vi "EditorEinfachCRIO-04-02-17.vi"() -> ()   [LabVIEW 2010]
panel:
  in  "Tab Control":T1(tab)
  in  "Dateiordner Housekeeping":path=path "C:/Users/Atmos/Desktop/Johnny"
  in  "Dateiname Housekeeping":string
  in  "DateiordnerECD1":path
  in  "DateinameECD1":string
  in  "DateiordnerECD2":path
  in  "DateinameECD2":string
  in  "Modul1/AI sicherer Bereich":dbl[][](array[numeric])=[[0.0, 0.0, 0.0, 0.0, 0.0, 0.0, 0.0, 0.0, 0.0, 0.0, 0.0, 0.0, 0.0, 0.0, 0.0, 0.0, 0.0, 0.0, 0.0, 0.0, 0.0, 0.0, 0.0, 0.0, 0.0, 0.0, 0.0, 0.0, 0.0, 0.0, 0.0, 0.0]]
  in  "Modul1/AIsNamen":string[](array[string])
  in  "Modul1/AI koeff":dbl[][](array[numeric])=[[0.0, 0.0, 0.0, 0.0, 0.0, 0.0, 0.0, 0.0, 0.0, 0.0, 0.0, 0.0, 0.0, 0.0, 0.0, 0.0, 0.0, 0.0, 0.0, 0.0, 0.0, 0.0, 0.0, 0.0, 0.0, 0.0, 0.0, 0.0, 0.0, 0.0, 0.0, 0.0]]
  in  "AIsNamenZurücksetzen":bool
  in  "Modul2/AIsNamen":string[](array[string])
  in  "Modul2/AI koeff":dbl[][](array[numeric])=[[0.0, 0.0, 0.0, 0.0, 0.0, 0.0, 0.0, 0.0, 0.0, 0.0, 0.0, 0.0, 0.0, 0.0, 0.0, 0.0, 0.0, 0.0, 0.0, 0.0, 0.0, 0.0, 0.0, 0.0, 0.0, 0.0, 0.0, 0.0, 0.0, 0.0, 0.0, 0.0]]
  in  "Modul2/AI sicherer Bereich":dbl[][](array[numeric])=[[0.0, 0.0, 0.0, 0.0, 0.0, 0.0, 0.0, 0.0, 0.0, 0.0, 0.0, 0.0, 0.0, 0.0, 0.0, 0.0, 0.0, 0.0, 0.0, 0.0, 0.0, 0.0, 0.0, 0.0, 0.0, 0.0, 0.0, 0.0, 0.0, 0.0, 0.0, 0.0]]
  in  "Modul3/AIsNamen":string[](array[string])
  in  "Modul3/AI koeff":dbl[][](array[numeric])=[[0.0, 0.0, 0.0, 0.0, 0.0, 0.0, 0.0, 0.0, 0.0, 0.0, 0.0, 0.0, 0.0, 0.0, 0.0, 0.0, 0.0, 0.0, 0.0, 0.0, 0.0, 0.0, 0.0, 0.0, 0.0, 0.0, 0.0, 0.0, 0.0, 0.0, 0.0, 0.0]]
  in  "Modul3/AI sicherer Bereich":dbl[][](array[numeric])=[[0.0, 0.0, 0.0, 0.0, 0.0, 0.0, 0.0, 0.0, 0.0, 0.0, 0.0, 0.0, 0.0, 0.0, 0.0, 0.0, 0.0, 0.0, 0.0, 0.0, 0.0, 0.0, 0.0, 0.0, 0.0, 0.0, 0.0, 0.0, 0.0, 0.0, 0.0, 0.0]]
  out "Schnelle Heizungen":string[](array[string])
  in  "Traps/MachsKoeff":dbl[][](array[numeric])=[[0.0, 0.0, 0.0, 0.0, 0.0, 0.0, 0.0, 0.0, 0.0, 0.0, 0.0, 0.0, 0.0, 0.0, 0.0, 0.0, 0.0, 0.0, 0.0, 0.0, 0.0, 0.0, 0.0, 0.0, 0.0, 0.0, 0.0, 0.0, 0.0, 0.0, 0.0, 0.0]]
  in  "Traps/Machs sicherer Bereich":dbl[][](array[numeric])=[[0.0, 0.0, 0.0, 0.0, 0.0, 0.0, 0.0, 0.0, 0.0, 0.0, 0.0, 0.0, 0.0, 0.0, 0.0, 0.0, 0.0, 0.0, 0.0, 0.0, 0.0, 0.0, 0.0, 0.0, 0.0, 0.0, 0.0, 0.0, 0.0, 0.0, 0.0, 0.0]]
  in  "LangsameHeizungen":string[](array[string])
  in  "ModuleLH":i32[](array[numeric]) min=1 max=3 step=1
  in  "AIsLH":i32[](array[numeric]) min=0 max=31 step=1
  in  "DIOsMod0Name":string[](array[string])
  in  "DIOsMod0Nr":i32[](array[numeric]) min=0 max=63 step=1
  in  "DIOsMod1Name":string[](array[string])
  in  "DIOsMod1Nr":i32[](array[numeric]) min=0 max=63 step=1
  in  "DIOsMod2AName":string[](array[string])
  in  "DIOsMod2ANr":i32[](array[numeric]) min=0 max=63 step=1
  in  "DIOsMod2BName":string[](array[string])
  in  "DIOsMod2BNr":i32[](array[numeric]) min=0 max=63 step=1
  out "AnzahlRegler/Modul":i32[](array[numeric])
  in  "Regler für den Probenfluß":i32
  in  "ReglerNameMod0":string[](array[string])
  in  "ReglerNameMod1":string[](array[string])
  in  "ReglerNameMod2A":string[](array[string])
  in  "ReglerNameMod2B":string[](array[string])
  in  "MWabfragenMod0":string[](array[string])=[":060F0401210120", ":06100401210120", ":06110401210120"]
  in  "MWabfragenMod1":string[](array[string])=[":060F0401210120", ":06100401210120", ":06110401210120"]
  in  "MWabfragenMod2A":string[](array[string])=[":060F0401210120", ":06100401210120", ":06110401210120"]
  in  "MWabfragenMod2B":string[](array[string])=[":060F0401210120", ":06100401210120", ":06110401210120"]
  in  "SPvorgebenMod0":string[](array[string])=[":060F020121", ":0610020121", ":0611020121"]
  in  "SPvorgebenMod1":string[](array[string])=[":060F020121", ":0610020121", ":0611020121"]
  in  "SPvorgebenMod2A":string[](array[string])=[":060F020121", ":0610020121", ":0611020121"]
  in  "SPvorgebenMod2B":string[](array[string])=[":060F020121", ":0610020121", ":0611020121"]
  in  "FaktorMod0":dbl[](array[numeric])=[9.375e-05, 9.375e-05, 9.375e-05]
  in  "FaktorMod1":dbl[](array[numeric])=[9.375e-05, 9.375e-05, 9.375e-05]
  in  "FaktorMod2A":dbl[](array[numeric])=[9.375e-05, 9.375e-05, 9.375e-05]
  in  "FaktorMod2B":dbl[](array[numeric])=[9.375e-05, 9.375e-05, 9.375e-05]
  in  "MWAntwortMod0":string[](array[string])=[":060F020121", ":0610020121", ":0611020121"]
  in  "MWAntwortMod1":string[](array[string])=[":060F020121", ":0610020121", ":0611020121"]
  in  "MWAntwortMod2A":string[](array[string])=[":060F020121", ":0610020121", ":0611020121"]
  in  "MWAntwortMod2B":string[](array[string])=[":060F020121", ":0610020121", ":0611020121"]
  in  "ReglerMod0 sicherer Bereich":dbl[][](array[numeric])=[[9.375e-05, 9.375e-05, 9.375e-05]]
  in  "ReglerMod1 sicherer Bereich":dbl[][](array[numeric])=[[9.375e-05, 9.375e-05, 9.375e-05]]
  in  "ReglerMod2A sicherer Bereich":dbl[][](array[numeric])=[[9.375e-05, 9.375e-05, 9.375e-05]]
  in  "ReglerMod2B sicherer Bereich":dbl[][](array[numeric])=[[9.375e-05, 9.375e-05, 9.375e-05]]
  in  "Metavariablen grüner Bereich":dbl[][](array[numeric])=[[0.0, 0.0, 0.0, 0.0, 0.0, 0.0, 0.0, 0.0, 0.0, 0.0, 0.0, 0.0, 0.0, 0.0, 0.0, 0.0, 0.0, 0.0, 0.0, 0.0, 0.0, 0.0, 0.0, 0.0, 0.0, 0.0, 0.0, 0.0, 0.0, 0.0, 0.0, 0.0]]
  in  "Metavariablen":string[](array[string])
  in  "Startmethode":i32=1
  in  "MethodeLöschen":bool
  in  "MethodeDuplizieren":bool
  out "Methoden":T2(array[cluster]) {"FPGAPID"."proportional gain (Kc)" format="%.11g"; "FPGAPID"."integral gain (Kc*Ts/Ti)" format="%.11g"; "FPGAPID"."derivative gain (Kc*Td/Ts)" format="%.11g"}
  in  "T_MainMach2":dbl[](array[numeric])
  in  "t_MainMach2":dbl[](array[numeric])
  in  "T_MainMach1":dbl[](array[numeric])
  in  "t_MainMach1":dbl[](array[numeric])
  in  "EinstellungenSpeichern":bool
  out "LangsameHeizungen":string[](array[string])
  in  "AllesSpeichern":bool
  in  "Methodenname":string
  in  "Int.Stop2":dbl
  in  "Int.Start2":dbl
  in  "Int.Stop1":dbl
  in  "Int.Start1":dbl
  in  "ZeitpktMS-2":dbl
  in  "ZeitpktMS-1":dbl
  in  "SPMPV":i32[](array[numeric])
  in  "ZeitpunkteMPV":dbl[](array[numeric])
  in  "Wert2":dbl
  in  "Vergleichsoperator2":dbl(ring) items=["<", "<=", "=", ">=", ">", "=/="]
  in  "AbfragbareVariablen2":dbl(ring) items=["T1-Trap1", "T1-Trap2", "T1-StirlingKühlkopf", "T1-PreCol1", "T1-PreCol2", "T1-MainCol1a", "T1-MainCol1b", "T1-MainCol2a", "T1-MainCol2b", "T1-Bronkhorst1a", "T1-Bronkhorst1b", "T1-Bronkhorst2a", "T1-Bronkhorst2b", "T1-2Pos1B", "T1-Spare9", "T1-2Pos1A", "T1-Spare10", "T1-TurboPump", "T1-StirlingPlatine", "T1-Spare5", "T1-Spare6", "T1-Spare7", "T1-Spare8", "F1-MFM1", "F1-MFM0D [mL]", "P1-MethaneHP", "P1-MethaneLP", "P1-Vacuum", "TurboSpeed", "I1-MS-AC", "I1-Trap1", "I1-Trap2", "T2-ECD1a", "T2-ECD1b", "T2-ECD2a", "T2-ECD2b", "T2-Col1a", "T2-Col1b", "T2-Col2a", "T2-Col2b", "T2-Spare1", "T2-Spare2", "T2-Oven_a", "T2-Oven_b", "T2-Spare3", "T2-Spare4", "T2-Spare5", "F2-MFM0", "F2-MFM2A", "F2-MFM2B", "P2-N2O_HP", "P2-N2O_LP", "P2-CO2_HP", "P2-CO2_LP", "AI-Spare1", "FL-MFM1000mL", "AI-Spare3", "AI-Spare4", "StirlingAlarm", "StirlingEmerg.", "AI-Spare7", "AI-Spare8", "AI-Spare9", "FL-MFM30mL", "T0-DC/DC5", "I0-24V_M0", "I0-48V_M1", "I0-24V_M1", "I0-28V_M2", "T0-Spare3", "T0-Spare2", "T0-Spare4", "T0-DC/DC7", "I0-20V_Laptop", "I0-28V_M1", "I0-24V_M2", "I0-12V_Licor", "T0-Spare1", "T0-Drier", "T0-Spare5", "F0-MFM0A [L]", "TL-Licor_a", "P0-Span-HP", "P0-spare1", "P0-Stickstoff-LP", "P0-Helium-LP", "P0-Cal-HP", "P0-P9Tavco[bar]", "F0-MFM0B [L]", "TL-Licor_b", "P0-Span-LP", "P0-spare2", "P0-Stickstoff-HP", "P0-Helium-HP", "P0-Cal-LP", "F0-MFM3", "T-Trap1", "T-Trap2", "T-PreMach1", "T-PreMach2", "T-MainMach1", "T-MainMach2", "PrC0", "PrC0-Licor", "PrC1-Säule2", "PrC1-Säule1", "MFC1-Sample", "MFC1-Methan", "PrC1-BackFlush1", "PrC1-BackFlush2", "MFC2A", "MFC2B", "MFC2C", "PrC2A", "MFC2D", "MFC2E", "PrC2B", "Gesamte Zeit", "Methodenzeit", "Zykluszeit Mod0", "Zykluszeit Mod1", "Zykluszeit Mod2A", "Zykluszeit Mod2B", "PositionMPV", "OverflowB", "OverflowA", "StirlingAlarmAlarm!"]
  in  "Dateien fürs MS schicken?":bool
  in  "Zwangsbedingungen":dbl[][](array[numeric])
  out "ZwangsBedingungen":string[][](array[string])
  in  "löschen":bool
  in  "Bedingung Nr. X":i32
  in  "Bedingung übernehmen":bool
  in  "Ausgangswert":dbl
  in  "BedienbareVariablen":dbl(ring) items=["D0-48V_M1", "D0-28V_M1", "D0-Pump2", "DL-LiCalS1H", "D-Spare2", "D-Spare4", "D0-28V_M2", "D0-Pump1", "D0-S01/EV1", "DL-Licor", "D0-EV3", "D0-EV2", "D1-StopMS", "D1-StartMS", "D1-TrapEvac1", "D1-TrapEvac2", "D1-2Pos1A", "D1-2Pos1B", "D1-TurboPump", "D1-PrePump", "D1-VacPump1", "D1-VacPump2", "D1-Stirling", "D1-P_MS", "D1-S1B(7)", "D1-S1A(6)", "D1-S1G", "D1-Fan3", "D1-LüfterMach1", "D1-LüfterMach2", "D1-MS-Power", "D2-SpülflußA", "D2-2Pos2B", "D2-2Pos2A", "D2-ECD1HeaterOff", "D2-Fan1", "D2-Fan2", "D2-Probe2A", "D2-Probe2B", "D2-SpülflußB", "D2-ECD2HeaterOff", "Servo1 an", "Servo2 an", "Servo1 kalt", "Servo2 kalt", "Heizen?Trap1", "Heizen?Trap2", "Heizen?PreCol1", "Heizen?PreCol2", "Heizen?MainCol1", "Heizen?MainCol2", "SollwertTrap1", "SollwertTrap2", "SollwertPreCol1", "SollwertPreCol2", "SollwertMainCol1", "SollwertMainCol2", "Methodennummer", "STOPP!!!", "H1-Valve1B heizen?", "H1-Bronkhorst1 heizen?", "H1-Bronkhorst2 heizen?", "H1-Valve1A heizen?", "H0-Drier heizen?", "HL-Licor heizen?", "H2-ECD2 heizen?", "H2-Oven heizen?", "H2-Spare1 heizen?", "H2-Col2 heizen?", "H2-Col1 heizen?", "H2-ECD1 heizen?", "H1-Valve1BSollwert", "H1-Bronkhorst1Sollwert", "H1-Bronkhorst2Sollwert", "H1-Valve1ASollwert", "H0-DrierSollwert", "HL-LicorSollwert", "H2-ECD2Sollwert", "H2-OvenSollwert", "H2-Spare1Sollwert", "H2-Col2Sollwert", "H2-Col1Sollwert", "H2-ECD1Sollwert", "PrC0", "PrC0-Licor", "PrC1-Säule2", "PrC1-Säule1", "MFC1-Sample", "MFC1-Methan", "PrC1-BackFlush1", "PrC1-BackFlush2", "MFC2A", "MFC2B", "MFC2C", "PrC2A", "MFC2D", "MFC2E", "PrC2B", "PositionMPV", "OverflowB", "OverflowA", "StirlingAlarmAlarm!"]
  in  "Wert1":dbl
  in  "Vergleichsoperator1":dbl(ring) items=["<", "<=", "=", ">=", ">", "=/="]
  in  "AbfragbareVariablen1":dbl(ring) items=["T1-Trap1", "T1-Trap2", "T1-StirlingKühlkopf", "T1-PreCol1", "T1-PreCol2", "T1-MainCol1a", "T1-MainCol1b", "T1-MainCol2a", "T1-MainCol2b", "T1-Bronkhorst1a", "T1-Bronkhorst1b", "T1-Bronkhorst2a", "T1-Bronkhorst2b", "T1-2Pos1B", "T1-Spare9", "T1-2Pos1A", "T1-Spare10", "T1-TurboPump", "T1-StirlingPlatine", "T1-Spare5", "T1-Spare6", "T1-Spare7", "T1-Spare8", "F1-MFM1", "F1-MFM0D [mL]", "P1-MethaneHP", "P1-MethaneLP", "P1-Vacuum", "TurboSpeed", "I1-MS-AC", "I1-Trap1", "I1-Trap2", "T2-ECD1a", "T2-ECD1b", "T2-ECD2a", "T2-ECD2b", "T2-Col1a", "T2-Col1b", "T2-Col2a", "T2-Col2b", "T2-Spare1", "T2-Spare2", "T2-Oven_a", "T2-Oven_b", "T2-Spare3", "T2-Spare4", "T2-Spare5", "F2-MFM0", "F2-MFM2A", "F2-MFM2B", "P2-N2O_HP", "P2-N2O_LP", "P2-CO2_HP", "P2-CO2_LP", "AI-Spare1", "FL-MFM1000mL", "AI-Spare3", "AI-Spare4", "StirlingAlarm", "StirlingEmerg.", "AI-Spare7", "AI-Spare8", "AI-Spare9", "FL-MFM30mL", "T0-DC/DC5", "I0-24V_M0", "I0-48V_M1", "I0-24V_M1", "I0-28V_M2", "T0-Spare3", "T0-Spare2", "T0-Spare4", "T0-DC/DC7", "I0-20V_Laptop", "I0-28V_M1", "I0-24V_M2", "I0-12V_Licor", "T0-Spare1", "T0-Drier", "T0-Spare5", "F0-MFM0A [L]", "TL-Licor_a", "P0-Span-HP", "P0-spare1", "P0-Stickstoff-LP", "P0-Helium-LP", "P0-Cal-HP", "P0-P9Tavco[bar]", "F0-MFM0B [L]", "TL-Licor_b", "P0-Span-LP", "P0-spare2", "P0-Stickstoff-HP", "P0-Helium-HP", "P0-Cal-LP", "F0-MFM3", "T-Trap1", "T-Trap2", "T-PreMach1", "T-PreMach2", "T-MainMach1", "T-MainMach2", "PrC0", "PrC0-Licor", "PrC1-Säule2", "PrC1-Säule1", "MFC1-Sample", "MFC1-Methan", "PrC1-BackFlush1", "PrC1-BackFlush2", "MFC2A", "MFC2B", "MFC2C", "PrC2A", "MFC2D", "MFC2E", "PrC2B", "Gesamte Zeit", "Methodenzeit", "Zykluszeit Mod0", "Zykluszeit Mod1", "Zykluszeit Mod2A", "Zykluszeit Mod2B", "PositionMPV", "OverflowB", "OverflowA", "StirlingAlarmAlarm!"]
  in  "Methode Nummer":i32
  in  "MethodeLaden":bool
  in  "EditorBeenden":bool
  in  "PIDs für \"träge\" Heizungen":T3(array[cluster])
  in  "T_PreMach2":dbl[](array[numeric])
  in  "t_PreMach2":dbl[](array[numeric])
  in  "T_PreMach1":dbl[](array[numeric])
  in  "t_PreMach1":dbl[](array[numeric])
  in  "SHSetpoints":dbl[][](array[numeric])
  in  "ZeitpktFPGAFixp":dbl[](array[numeric])
  in  "FPGAPID":T4(array[cluster]) {"proportional gain (Kc)" format="%.11g"; "integral gain (Kc*Ts/Ti)" format="%.11g"; "derivative gain (Kc*Td/Ts)" format="%.11g"}
  in  "ZeitpktFPGAPID":dbl[](array[numeric])
  in  "FPGABoolesch":bool[][](array[boolean])
  in  "ZPktFPGABoolesch":dbl[](array[numeric])
  in  "LHHeizen?":bool[](array[boolean])
  in  "LHSetpoints":dbl[](array[numeric])
  out "HorstMod1Name":string[](array[string])
  out "HorstMod2AName":string[](array[string])
  out "HorstMod2BName":string[](array[string])
  in  "HorstSPMod1":dbl[][](array[numeric])
  in  "HorstSPMod2A":dbl[][](array[numeric])
  in  "HorstSPMod2B":dbl[][](array[numeric])
  in  "Mod1HorstZeitpkt":dbl[](array[numeric])
  in  "Mod2AHorstZeitpkt":dbl[](array[numeric])
  in  "Mod2BHorstZeitpkt":dbl[](array[numeric])
  in  "HorstSPMod0":dbl[][](array[numeric])
  out "HorstMod0Name":string[](array[string])
  in  "Mod0HorstZeitpkt":dbl[](array[numeric])
  in  "DIOsSPMod2B":bool[][](array[boolean])
  in  "DIOsSPMod2A":bool[][](array[boolean])
  in  "DIOsSPMod1":bool[][](array[boolean])
  in  "ZeitpktDIOsMod2B":dbl[](array[numeric])
  in  "ZeitpktDIOsMod2A":dbl[](array[numeric])
  in  "ZeitpktDIOsMod1":dbl[](array[numeric])
  out "DIOsMod2BName":string[](array[string])
  out "DIOsMod2AName":string[](array[string])
  out "DIOsMod1Name":string[](array[string])
  out "DIOsMod0Name":string[](array[string])
  in  "DIOsSPMod0":bool[][](array[boolean])
  in  "ZeitpktDIOsMod0":dbl[](array[numeric])
  in  "MethodeSpeichern":bool
  in  "EinstellungenFertig":bool
  in  "Zykluslängen [s]":dbl[](array[numeric])
  # "Servo1         Servo2        Servo1        Servo2          Trap1          Trap2      PreMach1  PreMach2 MainMach1 MainMach2\n        an                 an              kalt             kalt            heizen         heizen        heizen         heizen         heizen         heizen"
  # "Trap1"
  # "Trap2"
  # "PreMach1"
  # "PreMach2"
  # "MainMach1"
  # "MainMach2"
  # "Sososo... alle Einstellungen vorgenommen? Wirklich alle? Sicher? Bereit, mit den Methoden fortzufahren? Na super, dann trau Dich und drück den Knopf!"
  # "Es können beliebig viele Methoden definiert werden; die gewünschte Nummer auswählen und die entsprechende Methode laden, dann nach Belieben dran rumfummeln und anschließend, wenns beliebt, die vorgenommenen Änderungen an der Methode übernehmen (das bedeutet NICHT, daß die Änderungen in einer Datei abgelegt werden, dafür gibts nen extra Knopp);\n\"Editor beenden\" dürfte klar sein. Und Tschüß!"
  # ":::Tom \"Awesome\"  Burner Jr.:::"
  # "Sollen die Daten vom MS abgefragt werden? Wenn ja, zu welchen Zeitpunkten (im Zyklus1)?"
  # "Schnelle Heizungen..."
  # "Die eingegebenen Punkte im (t-T)-Raum werden durch lineare Funktionen verbunden, jeweils definiert von Punkt zu Punkt."
  # "Stellung des Multipositionsventils; die Zeitpunkte beziehen sich auf den Zyklus von Modul0.\nDie Stellungen bezeichnen: \n1. Cal - 2. Span - 3. ? - 4. ? - \n5. Plank - 6. Air - 7. ?"
  # "Innerhalb welcher Zeitfenster (Modul1) soll der Probenfluß integriert werden?"
  # "Der Gipfel der Flexibilität: die Zwangsbedingungen!\nBitte boolesche Werte als 0/1 eingeben"
  # "Mod0\n\nMod1\n\nMod2A\n\nMod2B"
  # "UND"
  # "TSetpTrap1               TMaxTrap1              TSetpTrap2              TMaxTrap2             TMaxPreMach1      TMaxPreMach2        TMaxMainMach1      TMaxMainMach2"
  # "Dran denken: die Daten werden auf dem CRIO abgelegt, nicht auf dem ITX oder dem Notebook; Dateinamen bitte ohne Pfad und .tdms eingeben!"
  # "Die Analogeingänge sind entsprechend der AI-Module des CRIO angeordnet (3x32); es wird eine quadratische Kennlinie angenommen, also: y=a0+a1*x+a2*x^2;\ndie drei Koeffizienten werden in dieser Reihenfolge eingegeben (v.l.n.r.): a0, a1, a2. Die Alarmgrenzen werden folgendermaßen eingegeben: linke Spalte für untere Grenze, rechte Spalte für obere Grenze des sicheren Bereichs."
  # "Die Analogeingänge sind entsprechend der AI-Module des CRIO angeordnet (3x32); es wird eine quadratische Kennlinie angenommen, also: y=a0+a1*x+a2*x^2;\ndie drei Koeffizienten werden in dieser Reihenfolge eingegeben (v.l.n.r.): a0, a1, a2. Die Alarmgrenzen werden folgendermaßen eingegeben: linke Spalte für untere Grenze, rechte Spalte für obere Grenze des sicheren Bereichs."
  # "Die Analogeingänge sind entsprechend der AI-Module des CRIO angeordnet (3x32); es wird eine quadratische Kennlinie angenommen, also: y=a0+a1*x+a2*x^2;\ndie drei Koeffizienten werden in dieser Reihenfolge eingegeben (v.l.n.r.): a0, a1, a2. Die Alarmgrenzen werden folgendermaßen eingegeben: linke Spalte für untere Grenze, rechte Spalte für obere Grenze des sicheren Bereichs."
  # "Vorsicht!!! Wer hier nicht ganz genau weiß, was er tut, läßt bitte die Finger davon!\nDie Heizungen werden über den FPGA gesteuert, d.h. wenn man die Anzahl oder die Anschlüsse der Heizungen ändert, muß das FPGA-Programm entsprechend angepaßt werden.\nModuleLH bezieht sich auf die drei AI-Module des CRIO (1,2,3) und AIsLH auf den Anschluß im jeweiligen Modul."
  # "Die digitalen Ein-/Ausgänge werden modulweise aufgelistet (0, 1, 2A, 2B) und benannt; die zugehörigen Anschlüsse werden folgendermaßen durchgezählt: \nDIO 0...31 von Modul5 entspricht hier 0...31; DIO 0...31 von Modul6 entspricht hier 32+(0...31)=32...63."
  # "Die Bronkhorst-Regler werden modulweise zusammengefasst an den CRIO angeschlossen, Mod0 an Port0, Mod1 an Port1, Mod2A&2B an Port2;\ndie Strings für die Steuerung und Abfrage der Regler ergeben sich aus dem bronkhorstschen Handbuch; der Faktor berechnet sich durch \"Vollausschlag des Reglers (in der gewünschten Einheit, z.B. Bar)\"/32000;\n'Regler für den Probenfluß' meint die Nummer des entsprechenden Reglers in der Liste aller Regler, wobei der erste die Nummer 0 trägt."
  # "Wer will noch mehr, wer hat noch nichts? An dieser Stelle können weitere Variablen definiert werden, mit deren Hilfe die Zwangsbedingungen erst ihre volle Pracht und Mächtigkeit entfalten. Alle Variablen sind numerische Größen und haben damit beliebig viele Zustände. Beim Programmstart werden sie mit Null initialisiert.\nHöchschte Vorsicht ist beim Umbenennen oder gar Löschen von Variablen geboten, weil sich das fatal auf bestehende Zwangsbedingungen auswirken kann. Am besten immer nur neue Variablen hinzufügen, das garantiert sicheren Spaß ohne Spätfolgen."
  # "Im weiteren können beliebig viele Methoden definiert werden; mit welcher davon soll das Programm starten? Die erste Methode trägt die Nummer 0."
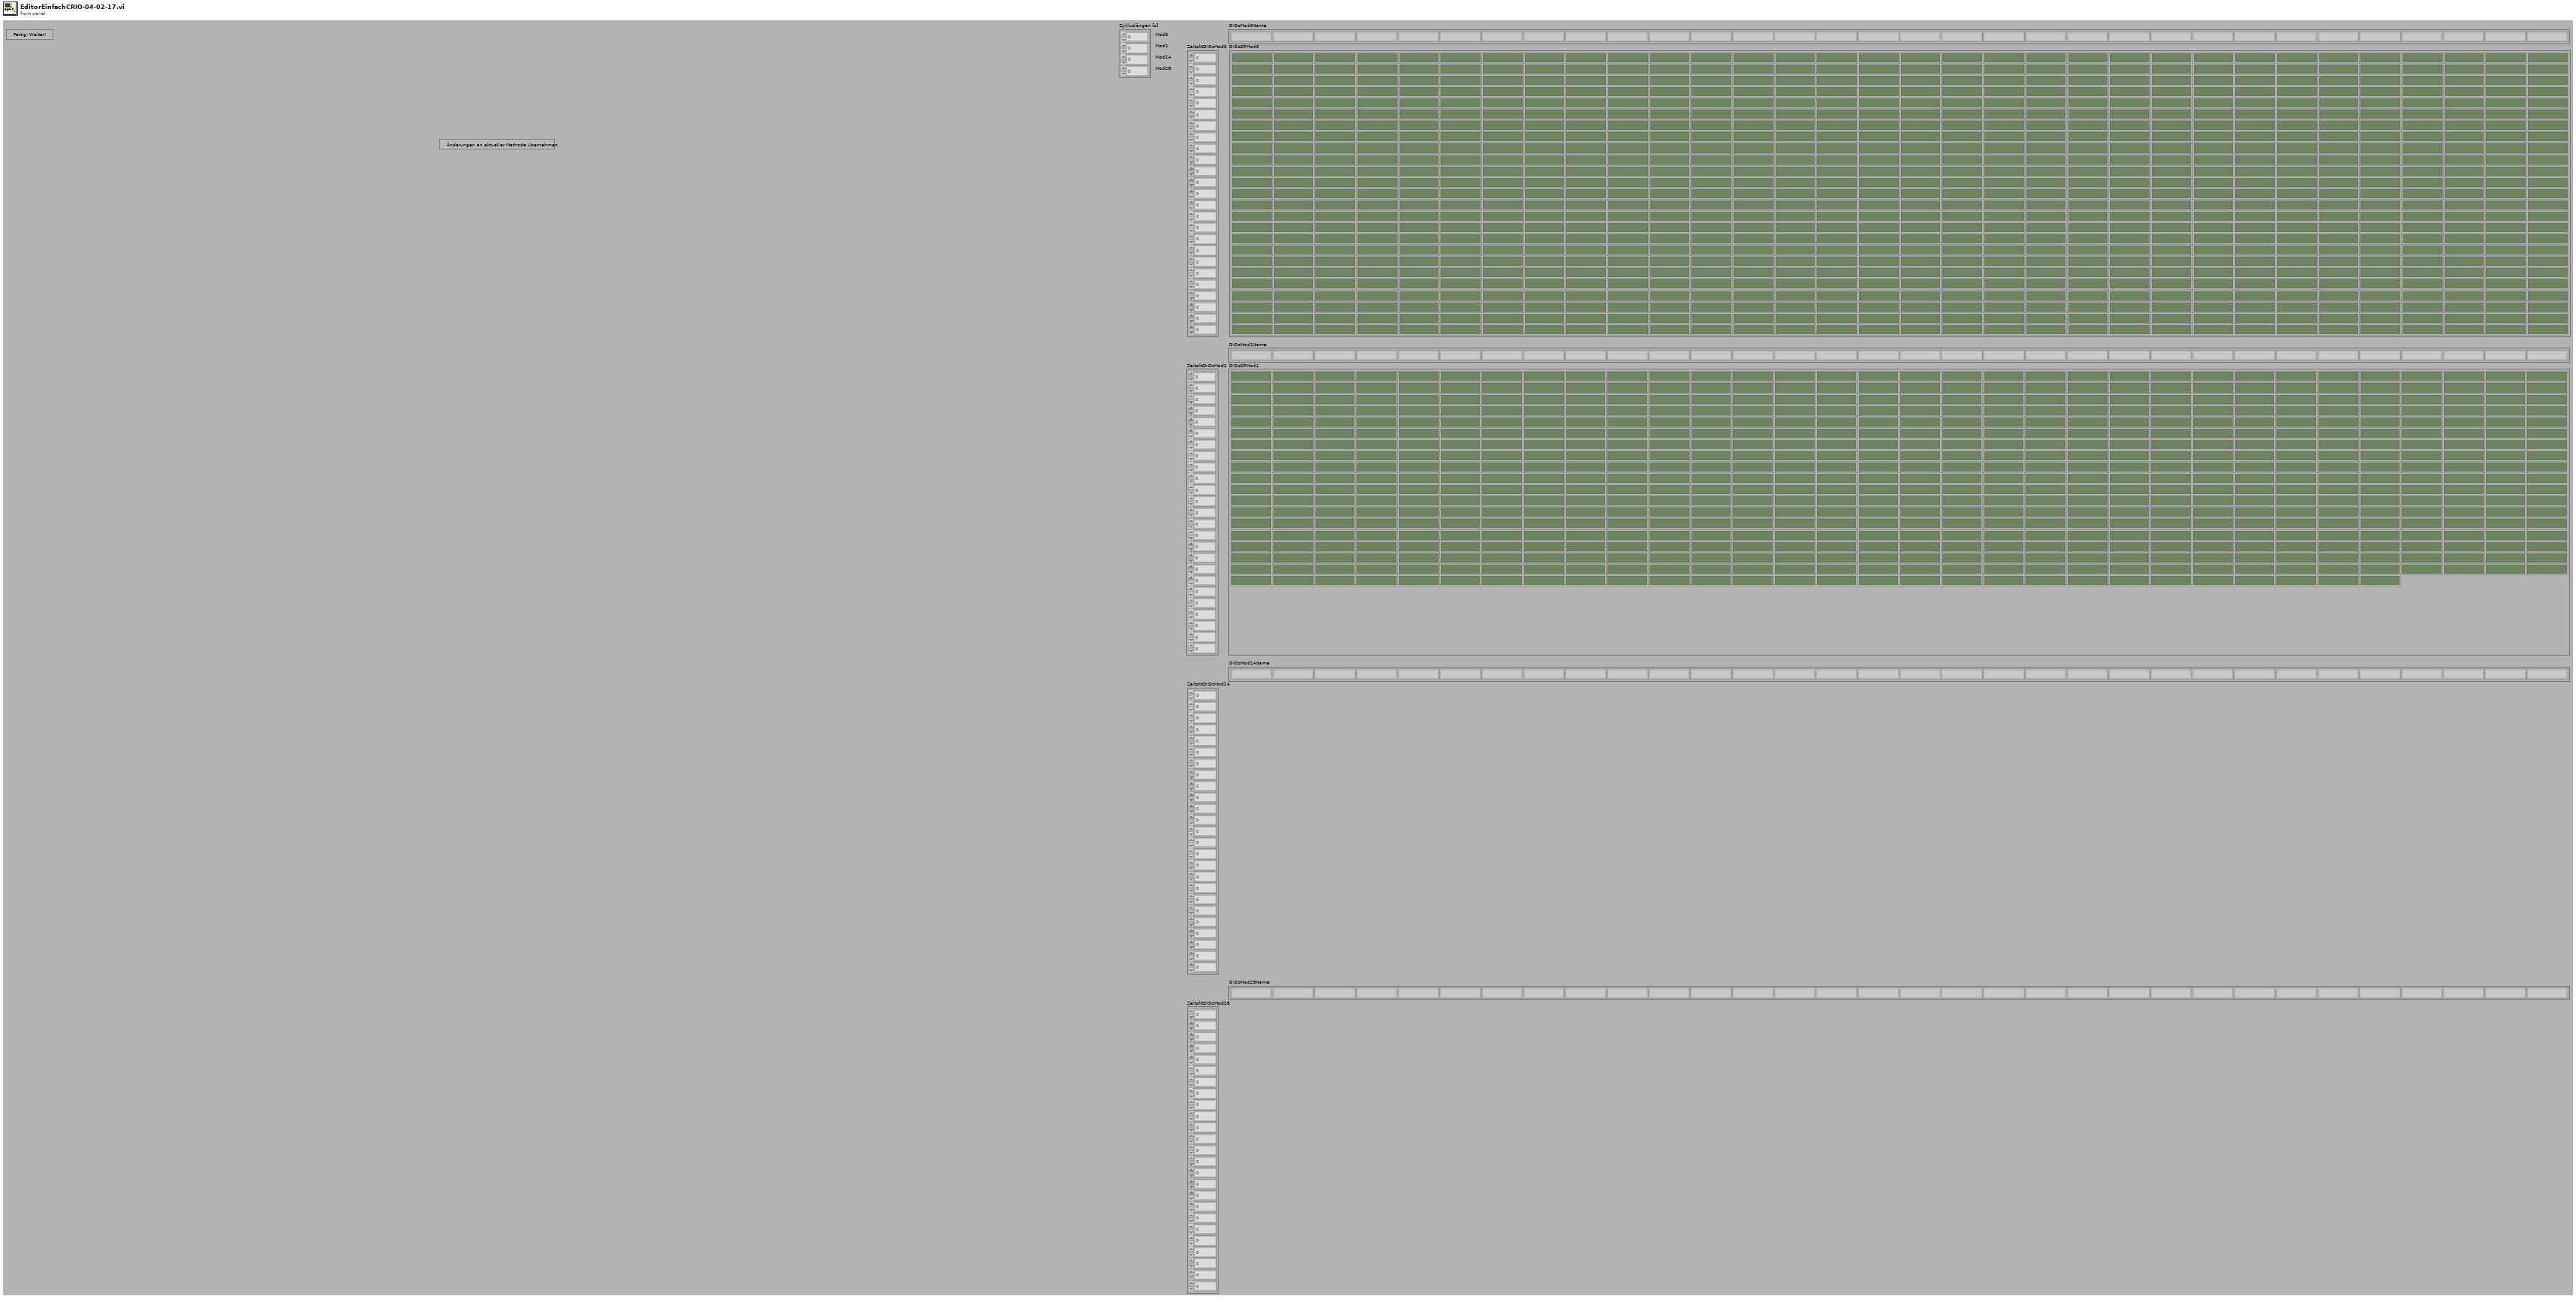
[diagram p1: front panel]
types:
  T1 = enum32{"Dateinamen", "Modul1/AIs", "Modul2/AIs", "Modul3/AIs", "schnelle Heizungen", "langsame Heizungen", "DIOs", "Horst-Regler", "Metavariablen", "Startmethode"}
  T2 = cluster{"Zykluslängen [s]":dbl[], "ZeitpktDIOsMod0":dbl[], "ZeitpktDIOsMod1":dbl[], "ZeitpktDIOsMod2A":dbl[], "ZeitpktDIOsMod2B":dbl[], "DIOsSPMod0":bool[][], "DIOsSPMod1":bool[][], "DIOsSPMod2A":bool[][], "DIOsSPMod2B":bool[][], "Mod0HorstZeitpkt":dbl[], "Mod1HorstZeitpkt":dbl[], "Mod2AHorstZeitpkt":dbl[], "Mod2BHorstZeitpkt":dbl[], "HorstSPMod0":dbl[][], "HorstSPMod1":dbl[][], "HorstSPMod2A":dbl[][], "HorstSPMod2B":dbl[][], "LHSetpoints":dbl[], "LHHeizen?":bool[], "ZPktFPGABoolesch":dbl[], "FPGABoolesch":bool[][], "ZeitpktFPGAPID":dbl[], "FPGAPID":cluster{"proportional gain (Kc)":fxp<+/-,16,8>, "integral gain (Kc*Ts/Ti)":fxp<+/-,16,8>, "derivative gain (Kc*Td/Ts)":fxp<+/-,16,8>}[][], "ZeitpktFPGAFixp":dbl[], "SHSetpoints":dbl[][], "t_PreMach1":dbl[], "T_PreMach1":dbl[], "t_PreMach2":dbl[], "T_PreMach2":dbl[], "PIDs für \"träge\" Heizungen":cluster{"proportional gain (Kc)":dbl, "integral time (Ti, min)":dbl, "derivative time (Td, min)":dbl}[], "Zwangsbedingungen":dbl[][], "Dateien fürs MS schicken?":bool, "ZeitpunkteMPV":dbl[], "SPMPV":i32[], "ZeitpktMS-1":dbl, "ZeitpktMS-2":dbl, "Int.Start1":dbl, "Int.Stop1":dbl, "Int.Start2":dbl, "Int.Stop2":dbl, "Methodenname":string, "t_MainMach1":dbl[], "T_MainMach1":dbl[], "t_MainMach2":dbl[], "T_MainMach2":dbl[]}[]
  T3 = cluster{"proportional gain (Kc)":dbl, "integral time (Ti, min)":dbl, "derivative time (Td, min)":dbl}[]
  T4 = cluster{"proportional gain (Kc)":fxp<+/-,16,8>, "integral gain (Kc*Ts/Ti)":fxp<+/-,16,8>, "derivative gain (Kc*Td/Ts)":fxp<+/-,16,8>}[][]
  T5 = cluster{"DIOsMod0Nr":i32[], "DIOsMod1Nr":i32[], "DIOsMod2ANr":i32[], "DIOsMod2BNr":i32[], "AIsLH":i32[], "AnzahlRegler/Modul":i32[], "Regler für den Probenfluß":i32, "SPvorgebenMod0":string[], "SPvorgebenMod1":string[], "SPvorgebenMod2A":string[], "SPvorgebenMod2B":string[], "MWAntwortMod0":string[], "MWAntwortMod1":string[], "MWAntwortMod2A":string[], "MWAntwortMod2B":string[], "FaktorMod0":dbl[], "FaktorMod1":dbl[], "FaktorMod2A":dbl[], "FaktorMod2B":dbl[], "MWabfragenMod0":string[], "MWabfragenMod1":string[], "MWabfragenMod2A":string[], "MWabfragenMod2B":string[], "Modul1/AI koeff":dbl[][], "Modul2/AI koeff":dbl[][], "Modul3/AI koeff":dbl[][], "Traps/MachsKoeff":dbl[][], "Modul1/AIsNamen":string[], "Modul2/AIsNamen":string[], "Modul3/AIsNamen":string[], "DIOsMod0Name":string[], "DIOsMod1Name":string[], "DIOsMod2AName":string[], "DIOsMod2BName":string[], "ReglerNameMod0":string[], "ReglerNameMod1":string[], "ReglerNameMod2A":string[], "ReglerNameMod2B":string[], "Startmethode":i32, "Dateiordner Housekeeping":path, "Dateiname Housekeeping":string, "DateiordnerECD1":path, "DateinameECD1":string, "DateiordnerECD2":path, "DateinameECD2":string, "LangsameHeizungen":string[], "ModuleLH":i32[], "Metavariablen":string[], "Modul1/AI sicherer Bereich":dbl[][], "Modul2/AI sicherer Bereich":dbl[][], "Modul3/AI sicherer Bereich":dbl[][], "Traps/Machs sicherer Bereich":dbl[][], "ReglerMod0 sicherer Bereich":dbl[][], "ReglerMod1 sicherer Bereich":dbl[][], "ReglerMod2A sicherer Bereich":dbl[][], "ReglerMod2B sicherer Bereich":dbl[][], "Metavariablen grüner Bereich":dbl[][]}
  T6 = enum16{"open", "replace", "create", "open or create", "replace or create", "replace or create with confirmation"}
  T7 = cluster{"Zykluslängen [s]":dbl[], "ZeitpktDIOsMod0":dbl[], "ZeitpktDIOsMod1":dbl[], "ZeitpktDIOsMod2A":dbl[], "ZeitpktDIOsMod2B":dbl[], "DIOsSPMod0":bool[][], "DIOsSPMod1":bool[][], "DIOsSPMod2A":bool[][], "DIOsSPMod2B":bool[][], "Mod0HorstZeitpkt":dbl[], "Mod1HorstZeitpkt":dbl[], "Mod2AHorstZeitpkt":dbl[], "Mod2BHorstZeitpkt":dbl[], "HorstSPMod0":dbl[][], "HorstSPMod1":dbl[][], "HorstSPMod2A":dbl[][], "HorstSPMod2B":dbl[][], "LHSetpoints":dbl[], "LHHeizen?":bool[], "ZPktFPGABoolesch":dbl[], "FPGABoolesch":bool[][], "ZeitpktFPGAPID":dbl[], "FPGAPID":cluster{"proportional gain (Kc)":fxp<+/-,16,8>, "integral gain (Kc*Ts/Ti)":fxp<+/-,16,8>, "derivative gain (Kc*Td/Ts)":fxp<+/-,16,8>}[][], "ZeitpktFPGAFixp":dbl[], "SHSetpoints":dbl[][], "t_PreMach1":dbl[], "T_PreMach1":dbl[], "t_PreMach2":dbl[], "T_PreMach2":dbl[], "PIDs für \"träge\" Heizungen":cluster{"proportional gain (Kc)":dbl, "integral time (Ti, min)":dbl, "derivative time (Td, min)":dbl}[], "Zwangsbedingungen":dbl[][], "Dateien fürs MS schicken?":bool, "ZeitpunkteMPV":dbl[], "SPMPV":i32[], "ZeitpktMS-1":dbl, "ZeitpktMS-2":dbl, "Int.Start1":dbl, "Int.Stop1":dbl, "Int.Start2":dbl, "Int.Stop2":dbl, "Methodenname":string, "t_MainMach1":dbl[], "T_MainMach1":dbl[], "t_MainMach2":dbl[], "T_MainMach2":dbl[]}
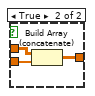
[diagram p9: hidden frame]
diagram:
  n1 = Open/Create/Replace File(file path (use dialog)=path "c:/einstellungen.perx" ("Dateipfad Einstellungen")) -> (refnum out=w20:refnum<file>, error out=w21:errorcluster)  [unwired: 5 in, 1 out]
  n2 = Read from Binary File(5:T5 {"DIOsMod0Nr"=[], "DIOsMod1Nr"=[], "DIOsMod2ANr"=[], "DIOsMod2BNr"=[], "AIsLH"=[], "AnzahlRegler/Modul"=[], "Regler für den Probenfluß"=0, "SPvorgebenMod0"=[], "SPvorgebenMod1"=[], "SPvorgebenMod2A"=[], "SPvorgebenMod2B"=[], "MWAntwortMod0"=[], "MWAntwortMod1"=[], "MWAntwortMod2A"=[], "MWAntwortMod2B"=[], "FaktorMod0"=[], "FaktorMod1"=[], "FaktorMod2A"=[], "FaktorMod2B"=[], "MWabfragenMod0"=[], "MWabfragenMod1"=[], "MWabfragenMod2A"=[], "MWabfragenMod2B"=[], "Modul1/AI koeff"=[], "Modul2/AI koeff"=[], "Modul3/AI koeff"=[], "Traps/MachsKoeff"=[], "Modul1/AIsNamen"=[], "Modul2/AIsNamen"=[], "Modul3/AIsNamen"=[], "DIOsMod0Name"=[], "DIOsMod1Name"=[], "DIOsMod2AName"=[], "DIOsMod2BName"=[], "ReglerNameMod0"=[], "ReglerNameMod1"=[], "ReglerNameMod2A"=[], "ReglerNameMod2B"=[], "Startmethode"=0, "Dateiordner Housekeeping"=path "", "Dateiname Housekeeping"="", "DateiordnerECD1"=path "", "DateinameECD1"="", "DateiordnerECD2"=path "", "DateinameECD2"="", "LangsameHeizungen"=[], "ModuleLH"=[], "Metavariablen"=[], "Modul1/AI sicherer Bereich"=[], "Modul2/AI sicherer Bereich"=[], "Modul3/AI sicherer Bereich"=[], "Traps/Machs sicherer Bereich"=[], "ReglerMod0 sicherer Bereich"=[], "ReglerMod1 sicherer Bereich"=[], "ReglerMod2A sicherer Bereich"=[], "ReglerMod2B sicherer Bereich"=[], "Metavariablen grüner Bereich"=[]} ("output cluster"), 8:w21, 11:w20) -> (0:w18:errorcluster, 2:w2:T5, 3:w19:refnum<file>)  [unwired: 3 in, 1 out]
  n3 = flat-sequence {
    tunnel: w2 -> [w96]
    tunnel: [w49] -> w7
    tunnel: [w119] -> w37
    tunnel: [w118] -> w36
    tunnel: [w117] -> w35
    tunnel: [w116] -> w34
    tunnel: [w115] -> w33
    tunnel: [w114] -> w32
    tunnel: [w113] -> w31
    tunnel: [w112] -> w30
    tunnel: [w111] -> w29
    tunnel: [w106] -> w28
    tunnel: [w105] -> w27
    tunnel: [w104] -> w26
    tunnel: [w103] -> w25
    tunnel: [w102] -> w24
    tunnel: [w101] -> w23
    tunnel: w16 -> [w100]
    tunnel: [w99] -> w8
    tunnel: w7 -> [w99]
    tunnel: [w98] -> w4
    tunnel: [w97] -> w3
    tunnel: w37 -> [w239]
    tunnel: w36 -> [w238]
    tunnel: w35 -> [w237]
    tunnel: w34 -> [w236]
    tunnel: w33 -> [w235]
    tunnel: w32 -> [w234]
    tunnel: w31 -> [w232]
    tunnel: w30 -> [w233]
    tunnel: w29 -> [w231]
    tunnel: w28 -> [w215]
    tunnel: w27 -> [w229]
    tunnel: w26 -> [w228]
    tunnel: w25 -> [w227]
    tunnel: w24 -> [w226]
    tunnel: w6 -> [w225]
    tunnel: w23 -> [w219]
    tunnel: w9 -> [w218]
    tunnel: w8 -> [w214]
    tunnel: w4 -> [w213]
    tunnel: w3 -> [w211]
    frame #0 {
      n4 = Unbundle(w96) -> ("DIOsMod0Nr"=w95:i32[], "DIOsMod1Nr"=w94:i32[], "DIOsMod2ANr"=w93:i32[], "DIOsMod2BNr"=w92:i32[], "AIsLH"=w91:i32[], "AnzahlRegler/Modul"=w90:i32[], "Regler für den Probenfluß"=w89:i32, "SPvorgebenMod0"=w88:string[], "SPvorgebenMod1"=w87:string[], "SPvorgebenMod2A"=w86:string[], "SPvorgebenMod2B"=w85:string[], "MWAntwortMod0"=w84:string[], "MWAntwortMod1"=w83:string[], "MWAntwortMod2A"=w82:string[], "MWAntwortMod2B"=w81:string[], "FaktorMod0"=w80:dbl[], "FaktorMod1"=w79:dbl[], "FaktorMod2A"=w78:dbl[], "FaktorMod2B"=w77:dbl[], "MWabfragenMod0"=w76:string[], "MWabfragenMod1"=w75:string[], "MWabfragenMod2A"=w74:string[], "MWabfragenMod2B"=w73:string[], "Modul1/AI koeff"=w72:dbl[][], "Modul2/AI koeff"=w71:dbl[][], "Modul3/AI koeff"=w70:dbl[][], "Traps/MachsKoeff"=w69:dbl[][], "Modul1/AIsNamen"=w68:string[], "Modul2/AIsNamen"=w67:string[], "Modul3/AIsNamen"=w66:string[], "DIOsMod0Name"=w65:string[], "DIOsMod1Name"=w64:string[], "DIOsMod2AName"=w63:string[], "DIOsMod2BName"=w62:string[], "ReglerNameMod0"=w61:string[], "ReglerNameMod1"=w60:string[], "ReglerNameMod2A"=w59:string[], "ReglerNameMod2B"=w58:string[], "Startmethode"=w57:i32, "Dateiordner Housekeeping"=w47:path, "Dateiname Housekeeping"=w56:string, "DateiordnerECD1"=w55:path, "DateinameECD1"=w54:string, "DateiordnerECD2"=w53:path, "DateinameECD2"=w52:string, "LangsameHeizungen"=w49:string[], "ModuleLH"=w50:i32[], "Metavariablen"=w48:string[], "Modul1/AI sicherer Bereich"=w46:dbl[][], "Modul2/AI sicherer Bereich"=w45:dbl[][], "Modul3/AI sicherer Bereich"=w44:dbl[][], "Traps/Machs sicherer Bereich"=w43:dbl[][], "ReglerMod0 sicherer Bereich"=w42:dbl[][], "ReglerMod1 sicherer Bereich"=w41:dbl[][], "ReglerMod2A sicherer Bereich"=w40:dbl[][], "ReglerMod2B sicherer Bereich"=w39:dbl[][], "Metavariablen grüner Bereich"=w38:dbl[][])
      n5 = property on="Modul1/AI sicherer Bereich" class="Arr (strict)"("Value"=w46) -> ()  [unwired: 2 in, 2 out]
      n6 = property on="Modul3/AI sicherer Bereich" class="Arr (strict)"("Value"=w44) -> ()  [unwired: 2 in, 2 out]
      n7 = property on="ReglerMod0 sicherer Bereich" class="Arr (strict)"("Value"=w42) -> ()  [unwired: 2 in, 2 out]
      n8 = property on="ReglerMod1 sicherer Bereich" class="Arr (strict)"("Value"=w41) -> ()  [unwired: 2 in, 2 out]
      n9 = property on="Modul2/AI sicherer Bereich" class="Arr (strict)"("Value"=w45) -> ()  [unwired: 2 in, 2 out]
      n10 = property on="Traps/Machs sicherer Bereich" class="Arr (strict)"("Value"=w43) -> ()  [unwired: 2 in, 2 out]
      n11 = property on="ReglerMod2A sicherer Bereich" class="Arr (strict)"("Value"=w40) -> ()  [unwired: 2 in, 2 out]
      n12 = property on="ReglerMod2B sicherer Bereich" class="Arr (strict)"("Value"=w39) -> ()  [unwired: 2 in, 2 out]
      n13 = property on="Metavariablen grüner Bereich" class="Arr (strict)"("Value"=w38) -> ()  [unwired: 2 in, 2 out]
      n14 = invoke on="MethodeLöschen" class="Bool (strict)" method="Reinit To Default"() -> ()  [unwired: 3 in, 3 out]
      n15 = property on="ModuleLH" class="Arr (strict)"("Value"=w50) -> ()  [unwired: 2 in, 2 out]
      n16 = property on="AIsLH" class="Arr (strict)"("Value"=w91) -> ()  [unwired: 2 in, 2 out]
      n17 = property on="Dateiname Housekeeping" class="Str"("Value"=w56) -> ()  [unwired: 2 in, 2 out]
      n18 = property on="DIOsMod0Nr" class="Arr (strict)"("Value"=w95) -> ()  [unwired: 2 in, 2 out]
      n19 = property on="DateiordnerECD1" class="Path"("Value"=w55) -> ()  [unwired: 2 in, 2 out]
      n20 = property on="DIOsMod1Nr" class="Arr (strict)"("Value"=w94) -> ()  [unwired: 2 in, 2 out]
      n21 = property on="DateinameECD1" class="Str"("Value"=w54) -> ()  [unwired: 2 in, 2 out]
      n22 = property on="DateiordnerECD2" class="Path"("Value"=w53) -> ()  [unwired: 2 in, 2 out]
      n23 = property on="DateinameECD2" class="Str"("Value"=w52) -> ()  [unwired: 2 in, 2 out]
      n24 = property on="DIOsMod2ANr" class="Arr (strict)"("Value"=w93) -> ()  [unwired: 2 in, 2 out]
      n25 = property on="LangsameHeizungen" class="Arr (strict)"("Value"=w49) -> ()  [unwired: 2 in, 2 out]
      n26 = property on="Metavariablen" class="Arr (strict)"("Value"=w48) -> ()  [unwired: 2 in, 2 out]
      n27 = property on="DIOsMod2BNr" class="Arr (strict)"("Value"=w92) -> ()  [unwired: 2 in, 2 out]
      n28 = property on="AnzahlRegler/Modul" class="Arr (strict)"("Value"=w90) -> ()  [unwired: 2 in, 2 out]
      n29 = property on="Regler für den Probenfluß" class="DigNum (strict)"("Value"=w89) -> ()  [unwired: 2 in, 2 out]
      n30 = property on="SPvorgebenMod0" class="Arr (strict)"("Value"=w88) -> ()  [unwired: 2 in, 2 out]
      n31 = property on="ReglerNameMod2B" class="Arr (strict)"("Value"=w58) -> ()  [unwired: 2 in, 2 out]
      n32 = property on="Startmethode" class="DigNum (strict)"("Value"=w57) -> ()  [unwired: 2 in, 2 out]
      n33 = property on="Dateiordner Housekeeping" class="Path"("Value"=w47) -> ()  [unwired: 2 in, 2 out]
      n34 = property on="SPvorgebenMod1" class="Arr (strict)"("Value"=w87) -> ()  [unwired: 2 in, 2 out]
      n35 = property on="SPvorgebenMod2A" class="Arr (strict)"("Value"=w86) -> ()  [unwired: 2 in, 2 out]
      n36 = property on="SPvorgebenMod2B" class="Arr (strict)"("Value"=w85) -> ()  [unwired: 2 in, 2 out]
      n37 = property on="MWAntwortMod0" class="Arr (strict)"("Value"=w84) -> ()  [unwired: 2 in, 2 out]
      n38 = property on="MWAntwortMod1" class="Arr (strict)"("Value"=w83) -> ()  [unwired: 2 in, 2 out]
      n39 = property on="MWAntwortMod2A" class="Arr (strict)"("Value"=w82) -> ()  [unwired: 2 in, 2 out]
      n40 = property on="MWAntwortMod2B" class="Arr (strict)"("Value"=w81) -> ()  [unwired: 2 in, 2 out]
      n41 = property on="FaktorMod0" class="Arr (strict)"("Value"=w80) -> ()  [unwired: 2 in, 2 out]
      n42 = property on="FaktorMod1" class="Arr (strict)"("Value"=w79) -> ()  [unwired: 2 in, 2 out]
      n43 = property on="FaktorMod2B" class="Arr (strict)"("Value"=w77) -> ()  [unwired: 2 in, 2 out]
      n44 = property on="MWabfragenMod0" class="Arr (strict)"("Value"=w76) -> ()  [unwired: 2 in, 2 out]
      n45 = property on="FaktorMod2A" class="Arr (strict)"("Value"=w78) -> ()  [unwired: 2 in, 2 out]
      n46 = property on="MWabfragenMod1" class="Arr (strict)"("Value"=w75) -> ()  [unwired: 2 in, 2 out]
      n47 = property on="MWabfragenMod2A" class="Arr (strict)"("Value"=w74) -> ()  [unwired: 2 in, 2 out]
      n48 = property on="MWabfragenMod2B" class="Arr (strict)"("Value"=w73) -> ()  [unwired: 2 in, 2 out]
      n49 = property on="Modul1/AI koeff" class="Arr (strict)"("Value"=w72) -> ()  [unwired: 2 in, 2 out]
      n50 = property on="Modul3/AI koeff" class="Arr (strict)"("Value"=w70) -> ()  [unwired: 2 in, 2 out]
      n51 = property on="Traps/MachsKoeff" class="Arr (strict)"("Value"=w69) -> ()  [unwired: 2 in, 2 out]
      n52 = property on="Modul1/AIsNamen" class="Arr (strict)"("Value"=w68) -> ()  [unwired: 2 in, 2 out]
      n53 = property on="Modul2/AIsNamen" class="Arr (strict)"("Value"=w67) -> ()  [unwired: 2 in, 2 out]
      n54 = property on="Modul3/AIsNamen" class="Arr (strict)"("Value"=w66) -> ()  [unwired: 2 in, 2 out]
      n55 = property on="Modul2/AI koeff" class="Arr (strict)"("Value"=w71) -> ()  [unwired: 2 in, 2 out]
      n56 = property on="DIOsMod0Name" class="Arr (strict)"("Value"=w65) -> ()  [unwired: 2 in, 2 out]
      n57 = property on="DIOsMod1Name" class="Arr (strict)"("Value"=w64) -> ()  [unwired: 2 in, 2 out]
      n58 = property on="DIOsMod2AName" class="Arr (strict)"("Value"=w63) -> ()  [unwired: 2 in, 2 out]
      n59 = property on="DIOsMod2BName" class="Arr (strict)"("Value"=w62) -> ()  [unwired: 2 in, 2 out]
      n60 = property on="ReglerNameMod0" class="Arr (strict)"("Value"=w61) -> ()  [unwired: 2 in, 2 out]
      n61 = property on="ReglerNameMod1" class="Arr (strict)"("Value"=w60) -> ()  [unwired: 2 in, 2 out]
      n62 = property on="ReglerNameMod2A" class="Arr (strict)"("Value"=w59) -> ()  [unwired: 2 in, 2 out]
      "Schnelle Heizungen" <- string[] ["Trap1 [°C]", "Trap2 [°C]", "PreCol1 [°C]", "PreCol2 [°C]", "MainCol1 [°C]", "MainCol2 [°C]"]
    }
    frame #1 {
      n63 = while {
        tunnel: ["DIOsMod0Name"] -> w119
        tunnel: ["DIOsMod1Name"] -> w118
        tunnel: ["DIOsMod2AName"] -> w117
        tunnel: ["DIOsMod2BName"] -> w116
        tunnel: ["ReglerNameMod0"] -> w115
        tunnel: ["ReglerNameMod1"] -> w114
        tunnel: ["ReglerNameMod2A"] -> w113
        tunnel: ["ReglerNameMod2B"] -> w112
        tunnel: [w137] -> w111
        tunnel: ["ReglerNameMod2B"] -> w110
        tunnel: ["ReglerNameMod2A"] -> w109
        tunnel: ["ReglerNameMod1"] -> w108
        tunnel: ["ReglerNameMod0"] -> w107
        tunnel: ["DIOsMod0Name"] -> w105
        tunnel: ["DIOsMod1Name"] -> w104
        tunnel: ["DIOsMod2AName"] -> w103
        tunnel: ["DIOsMod2BName"] -> w102
        tunnel: ["LangsameHeizungen"] -> w101
        tunnel: w100 -> [w132]
        tunnel: ["Metavariablen"] -> w98
        tunnel: ["Metavariablen"] -> w97
        stop <- "EinstellungenFertig" stop-if-true
        n64 = Wait (ms)(milliseconds to wait=u32 500 ("Zu wartende ms")) -> ()  [unwired: 1 out]
        n65 = case shown="True" "AIsNamenZurücksetzen" {
          frame False {
          }
          frame True {
            w203 = 32 ("Länge")
            w204 = string[] ["Mod1/AI0", "Mod1/AI1", "Mod1/AI2", "Mod1/AI3", "Mod1/AI4", "Mod1/AI5", "Mod1/AI6", "Mod1/AI7", "Mod1/AI8", "Mod1/AI9", "Mod1/AI10", "Mod1/AI11", "Mod1/AI12", "Mod1/AI13", "Mod1/AI14", "Mod1/AI15", "Mod1/AI16", "Mod1/AI17", "Mod1/AI18", "Mod1/AI19", "Mod1/AI20", "Mod1/AI21", "Mod1/AI22", "Mod1/AI23", "Mod1/AI24", "Mod1/AI25", "Mod1/AI26", "Mod1/AI27", "Mod1/AI28", "Mod1/AI29", "Mod1/AI30", "Mod1/AI31", "Mod2/AI0", "Mod2/AI1", "Mod2/AI2", "Mod2/AI3", "Mod2/AI4", "Mod2/AI5", "Mod2/AI6", "Mod2/AI7", "Mod2/AI8", "Mod2/AI9", "Mod2/AI10", "Mod2/AI11", "Mod2/AI12", "Mod2/AI13", "Mod2/AI14", "Mod2/AI15", "Mod2/AI16", "Mod2/AI17", "Mod2/AI18", "Mod2/AI19", "Mod2/AI20", "Mod2/AI21", "Mod2/AI22", "Mod2/AI23", "Mod2/AI24", "Mod2/AI25", "Mod2/AI26", "Mod2/AI27", "Mod2/AI28", "Mod2/AI29", "Mod2/AI30", "Mod2/AI31", "Mod3/AI0", "Mod3/AI1", "Mod3/AI2", "Mod3/AI3", "Mod3/AI4", "Mod3/AI5", "Mod3/AI6", "Mod3/AI7", "Mod3/AI8", "Mod3/AI9", "Mod3/AI10", "Mod3/AI11", "Mod3/AI12", "Mod3/AI13", "Mod3/AI14", "Mod3/AI15", "Mod3/AI16", "Mod3/AI17", "Mod3/AI18", "Mod3/AI19", "Mod3/AI20", "Mod3/AI21", "Mod3/AI22", "Mod3/AI23", "Mod3/AI24", "Mod3/AI25", "Mod3/AI26", "Mod3/AI27", "Mod3/AI28", "Mod3/AI29", "Mod3/AI30", "Mod3/AI31"] ("Array 2")
            n66 = Array Subset(array=w204, index=32 ("Index"), length=w203) -> (w200:string[])
            n67 = Array Subset(array=w204, index=0 ("Index"), length=w203) -> (w201:string[])
            n68 = Array Subset(array=w204, index=64 ("Index"), length=w203) -> (w199:string[])
            n69 = local write "Modul2/AIsNamen"(w200) -> ()
            n70 = local write "Modul1/AIsNamen"(w201) -> ()
            n71 = local write "Modul3/AIsNamen"(w199) -> ()
          }
        }
        n72 = Array Size(array="ReglerNameMod0") -> (size(s)=w187:i32)
        n73 = Array Size(array="ReglerNameMod1") -> (size(s)=w186:i32)
        n74 = Array Size(array="ReglerNameMod2A") -> (size(s)=w185:i32)
        n75 = Array Size(array="ReglerNameMod2B") -> (size(s)=w184:i32)
        n76 = Build Array "Anzahl Horst/Modul"(w187, w186, w185, w184) -> (w136:i32[])
        n77 = flat-sequence {
          tunnel: w136 -> [w197]
          tunnel: [w198] -> w135
          frame #0 {
            "AnzahlRegler/Modul" <- w197
          }
          frame #1 {
            n78 = local read "AnzahlRegler/Modul"() -> (w198:i32[])
          }
        }
        n79 = Build Array (concatenate)("Modul1/AIsNamen", "Modul2/AIsNamen", "Modul3/AIsNamen") -> (w137:string[])
        n80 = Bundle("DIOsMod0Nr"="DIOsMod0Nr", "DIOsMod1Nr"="DIOsMod1Nr", "DIOsMod2ANr"="DIOsMod2ANr", "DIOsMod2BNr"="DIOsMod2BNr", "AIsLH"="AIsLH", "AnzahlRegler/Modul"=w135, "Regler für den Probenfluß"="Regler für den Probenfluß", "SPvorgebenMod0"="SPvorgebenMod0", "SPvorgebenMod1"="SPvorgebenMod1", "SPvorgebenMod2A"="SPvorgebenMod2A", "SPvorgebenMod2B"="SPvorgebenMod2B", "MWAntwortMod0"="MWAntwortMod0", "MWAntwortMod1"="MWAntwortMod1", "MWAntwortMod2A"="MWAntwortMod2A", "MWAntwortMod2B"="MWAntwortMod2B", "FaktorMod0"="FaktorMod0", "FaktorMod1"="FaktorMod1", "FaktorMod2A"="FaktorMod2A", "FaktorMod2B"="FaktorMod2B", "MWabfragenMod0"="MWabfragenMod0", "MWabfragenMod1"="MWabfragenMod1", "MWabfragenMod2A"="MWabfragenMod2A", "MWabfragenMod2B"="MWabfragenMod2B", "Modul1/AI koeff"="Modul1/AI koeff", "Modul2/AI koeff"="Modul2/AI koeff", "Modul3/AI koeff"="Modul3/AI koeff", "Traps/MachsKoeff"="Traps/MachsKoeff", "Modul1/AIsNamen"="Modul1/AIsNamen", "Modul2/AIsNamen"="Modul2/AIsNamen", "Modul3/AIsNamen"="Modul3/AIsNamen", "DIOsMod0Name"="DIOsMod0Name", "DIOsMod1Name"="DIOsMod1Name", "DIOsMod2AName"="DIOsMod2AName", "DIOsMod2BName"="DIOsMod2BName", "ReglerNameMod0"="ReglerNameMod0", "ReglerNameMod1"="ReglerNameMod1", "ReglerNameMod2A"="ReglerNameMod2A", "ReglerNameMod2B"="ReglerNameMod2B", "Startmethode"="Startmethode", "Dateiordner Housekeeping"="Dateiordner Housekeeping", "Dateiname Housekeeping"="Dateiname Housekeeping", "DateiordnerECD1"="DateiordnerECD1", "DateinameECD1"="DateinameECD1", "DateiordnerECD2"="DateiordnerECD2", "DateinameECD2"="DateinameECD2", "LangsameHeizungen"="LangsameHeizungen", "ModuleLH"="ModuleLH", "Metavariablen"="Metavariablen", "Modul1/AI sicherer Bereich"="Modul1/AI sicherer Bereich", "Modul2/AI sicherer Bereich"="Modul2/AI sicherer Bereich", "Modul3/AI sicherer Bereich"="Modul3/AI sicherer Bereich", "Traps/Machs sicherer Bereich"="Traps/Machs sicherer Bereich", "ReglerMod0 sicherer Bereich"="ReglerMod0 sicherer Bereich", "ReglerMod1 sicherer Bereich"="ReglerMod1 sicherer Bereich", "ReglerMod2A sicherer Bereich"="ReglerMod2A sicherer Bereich", "ReglerMod2B sicherer Bereich"="ReglerMod2B sicherer Bereich", "Metavariablen grüner Bereich"="Metavariablen grüner Bereich") -> (w131:T5)  [unwired: 1 in]
        n81 = case shown="True" "EinstellungenSpeichern" {
          tunnel: w132 -> [_ _]
          tunnel: w131 -> [_ w193]
          frame False {
          }
          frame True {
            n82 = Open/Create/Replace File(file path (use dialog)=path "c:/einstellungen.perx" ("Dateipfad Einstellungen"), operation (0:open)=T6."replace or create" ("Operation (0:Öffnen)")) -> (refnum out=w195:refnum<file>, error out=w192:errorcluster)  [unwired: 4 in, 1 out]
            n83 = Write to Binary File(file (use dialog)=w195, data=w193, error in=w192) -> (refnum out=w194:refnum<file>, error out=w191:errorcluster)  [unwired: 3 in, 1 out]
            n84 = Close File(refnum=w194, error in=w191) -> (error out=w190:errorcluster)  [unwired: 1 out]
            n85 = call <vilib>:"Simple Error Handler.vi"("error in (no error)"=w190) -> ()  [unwired: 4 in, 5 out]
          }
        }
      }
      n86 = Build Array (concatenate)(w107, w108, w109, w110) -> (w106:string[])
    }
    frame #2 {
      w220 = string[] ["<", "<=", "=", ">=", ">", "=/="] ("Strings []")
      n87 = for {
        tunnel: w214 -> [w241] mode=indexing
        tunnel: [w243] -> w209 mode=indexing
        tunnel: [w240] -> w208 mode=indexing
        n88 = Concatenate Strings(w241, " heizen?" ("String")) -> (w243:string)
        n89 = Concatenate Strings(w241, "Sollwert" ("String")) -> (w240:string)
      }
      n90 = Build Array (concatenate)(w229, w228, w227, w226) -> (w224:string[])
      n91 = Build Array (concatenate)(w209, w208) -> (w207:string[])
      n92 = Build Array (concatenate)(w224, string[] ["Servo1 an", "Servo2 an", "Servo1 kalt", "Servo2 kalt", "Heizen?Trap1", "Heizen?Trap2", "Heizen?PreCol1", "Heizen?PreCol2", "Heizen?MainCol1", "Heizen?MainCol2", "SollwertTrap1", "SollwertTrap2", "SollwertPreCol1", "SollwertPreCol2", "SollwertMainCol1", "SollwertMainCol2", "Methodennummer", "STOPP!!!"], w207, w215, "PositionMPV", w211) -> (w222:string[])
      n93 = Build Array (concatenate)(w231, string[] ["T-Trap1", "T-Trap2", "T-PreMach1", "T-PreMach2", "T-MainMach1", "T-MainMach2"], w215, string[] ["Gesamte Zeit", "Methodenzeit", "Zykluszeit Mod0", "Zykluszeit Mod1", "Zykluszeit Mod2A", "Zykluszeit Mod2B"] ("Array"), "PositionMPV", w213) -> (w221:string[])
      n94 = property on="Vergleichsoperator2" class="Ring (strict)"("Strings []"=w220) -> ()  [unwired: 2 in, 2 out]
      n95 = while {
        tunnel: w239 -> [w313]
        tunnel: w238 -> [w312]
        tunnel: w237 -> [w311]
        tunnel: w236 -> [w310]
        tunnel: w235 -> [w309]
        tunnel: w234 -> [w308]
        tunnel: w233 -> [w307]
        tunnel: w232 -> [w306]
        shift-right: [w265] -> w216
        shift-left: w225 -> [w247]
        tunnel: w221 -> [w272]
        tunnel: w220 -> [w271]
        tunnel: w222 -> [w270]
        tunnel: w218 -> [w264]
        stop <- w303 stop-if-true
        n96 = Index Array(array=w247, index="Methode Nummer") -> (element=w302:T7)
        n97 = Unbundle(w302) -> ("Zykluslängen [s]"=w301:dbl[], "ZeitpktDIOsMod0"=w300:dbl[], "ZeitpktDIOsMod1"=w299:dbl[], "ZeitpktDIOsMod2A"=w298:dbl[], "ZeitpktDIOsMod2B"=w297:dbl[], "DIOsSPMod0"=w296:bool[][], "DIOsSPMod1"=w295:bool[][], "DIOsSPMod2A"=w294:bool[][], "DIOsSPMod2B"=w293:bool[][], "Mod0HorstZeitpkt"=w292:dbl[], "Mod1HorstZeitpkt"=w291:dbl[], "Mod2AHorstZeitpkt"=w290:dbl[], "Mod2BHorstZeitpkt"=w289:dbl[], "HorstSPMod0"=w288:dbl[][], "HorstSPMod1"=w287:dbl[][], "HorstSPMod2A"=w286:dbl[][], "HorstSPMod2B"=w285:dbl[][], "LHSetpoints"=w284:dbl[], "LHHeizen?"=w283:bool[], "ZPktFPGABoolesch"=w282:dbl[], "FPGABoolesch"=w281:bool[][], "ZeitpktFPGAPID"=w280:dbl[], "FPGAPID"=w279:T4, "ZeitpktFPGAFixp"=w278:dbl[], "SHSetpoints"=w277:dbl[][], "t_PreMach1"=w276:dbl[], "T_PreMach1"=w275:dbl[], "t_PreMach2"=w274:dbl[], "T_PreMach2"=w273:dbl[], "PIDs für \"träge\" Heizungen"=w269:T3, "Zwangsbedingungen"=w268:dbl[][], "Dateien fürs MS schicken?"=w267:bool, "ZeitpunkteMPV"=w260:dbl[], "SPMPV"=w259:i32[], "ZeitpktMS-1"=w262:dbl, "ZeitpktMS-2"=w261:dbl, "Int.Start1"=w258:dbl, "Int.Stop1"=w257:dbl, "Int.Start2"=w256:dbl, "Int.Stop2"=w255:dbl, "Methodenname"=w263:string, "t_MainMach1"=w254:dbl[], "T_MainMach1"=w253:dbl[], "t_MainMach2"=w252:dbl[], "T_MainMach2"=w251:dbl[])
        n98 = property on="LHHeizen?" class="Arr (strict)"("Value"=w283) -> ()  [unwired: 2 in, 2 out]
        n99 = property on="FPGAPID" class="Arr (strict)"("Value"=w279) -> ()  [unwired: 2 in, 2 out]
        n100 = property on="SPMPV" class="Arr (strict)"("Value"=w259) -> ()  [unwired: 2 in, 2 out]
        n101 = property on="Int.Start1" class="DigNum (strict)"("Value"=w258) -> ()  [unwired: 2 in, 2 out]
        n102 = property on="Int.Stop1" class="DigNum (strict)"("Value"=w257) -> ()  [unwired: 2 in, 2 out]
        n103 = property on="Int.Start2" class="DigNum (strict)"("Value"=w256) -> ()  [unwired: 2 in, 2 out]
        n104 = property on="Int.Stop2" class="DigNum (strict)"("Value"=w255) -> ()  [unwired: 2 in, 2 out]
        n105 = property on="T_MainMach2" class="Arr (strict)"("Value"=w251) -> ()  [unwired: 2 in, 2 out]
        n106 = property on="Zykluslängen [s]" class="Arr (strict)"("Value"=w301) -> ()  [unwired: 2 in, 2 out]
        n107 = property on="ZeitpktDIOsMod0" class="Arr (strict)"("Value"=w300) -> ()  [unwired: 2 in, 2 out]
        n108 = property on="Mod2BHorstZeitpkt" class="Arr (strict)"("Value"=w289) -> ()  [unwired: 2 in, 2 out]
        n109 = property on="HorstSPMod0" class="Arr (strict)"("Value"=w288) -> ()  [unwired: 2 in, 2 out]
        n110 = property on="LHSetpoints" class="Arr (strict)"("Value"=w284) -> ()  [unwired: 2 in, 2 out]
        n111 = property on="ZPktFPGABoolesch" class="Arr (strict)"("Value"=w282) -> ()  [unwired: 2 in, 2 out]
        n112 = property on="FPGABoolesch" class="Arr (strict)"("Value"=w281) -> ()  [unwired: 2 in, 2 out]
        n113 = property on="T_PreMach2" class="Arr (strict)"("Value"=w273) -> ()  [unwired: 2 in, 2 out]
        n114 = property on="PIDs für \"träge\" Heizungen" class="Arr (strict)"("Value"=w269) -> ()  [unwired: 2 in, 2 out]
        n115 = property on="DIOsSPMod1" class="Arr (strict)"("Value"=w295) -> ()  [unwired: 2 in, 2 out]
        n116 = property on="DIOsSPMod2A" class="Arr (strict)"("Value"=w294) -> ()  [unwired: 2 in, 2 out]
        n117 = property on="HorstSPMod1" class="Arr (strict)"("Value"=w287) -> ()  [unwired: 2 in, 2 out]
        n118 = property on="HorstSPMod2A" class="Arr (strict)"("Value"=w286) -> ()  [unwired: 2 in, 2 out]
        n119 = property on="HorstSPMod2B" class="Arr (strict)"("Value"=w285) -> ()  [unwired: 2 in, 2 out]
        n120 = property on="ZeitpktFPGAPID" class="Arr (strict)"("Value"=w280) -> ()  [unwired: 2 in, 2 out]
        n121 = property on="ZeitpktFPGAFixp" class="Arr (strict)"("Value"=w278) -> ()  [unwired: 2 in, 2 out]
        n122 = property on="SHSetpoints" class="Arr (strict)"("Value"=w277) -> ()  [unwired: 2 in, 2 out]
        n123 = property on="t_PreMach1" class="Arr (strict)"("Value"=w276) -> ()  [unwired: 2 in, 2 out]
        n124 = property on="T_PreMach1" class="Arr (strict)"("Value"=w275) -> ()  [unwired: 2 in, 2 out]
        n125 = property on="t_PreMach2" class="Arr (strict)"("Value"=w274) -> ()  [unwired: 2 in, 2 out]
        n126 = property on="ZeitpktDIOsMod1" class="Arr (strict)"("Value"=w299) -> ()  [unwired: 2 in, 2 out]
        n127 = property on="ZeitpktDIOsMod2A" class="Arr (strict)"("Value"=w298) -> ()  [unwired: 2 in, 2 out]
        n128 = property on="ZeitpktDIOsMod2B" class="Arr (strict)"("Value"=w297) -> ()  [unwired: 2 in, 2 out]
        n129 = property on="DIOsSPMod0" class="Arr (strict)"("Value"=w296) -> ()  [unwired: 2 in, 2 out]
        n130 = property on="DIOsSPMod2B" class="Arr (strict)"("Value"=w293) -> ()  [unwired: 2 in, 2 out]
        n131 = property on="Mod0HorstZeitpkt" class="Arr (strict)"("Value"=w292) -> ()  [unwired: 2 in, 2 out]
        n132 = property on="Mod1HorstZeitpkt" class="Arr (strict)"("Value"=w291) -> ()  [unwired: 2 in, 2 out]
        n133 = property on="Mod2AHorstZeitpkt" class="Arr (strict)"("Value"=w290) -> ()  [unwired: 2 in, 2 out]
        n134 = property on="Dateien fürs MS schicken?" class="Bool (strict)"("Value"=w267) -> ()  [unwired: 2 in, 2 out]
        n135 = property on="ZeitpunkteMPV" class="Arr (strict)"("Value"=w260) -> ()  [unwired: 2 in, 2 out]
        n136 = property on="ZeitpktMS-1" class="DigNum (strict)"("Value"=w262) -> ()  [unwired: 2 in, 2 out]
        n137 = property on="ZeitpktMS-2" class="DigNum (strict)"("Value"=w261) -> ()  [unwired: 2 in, 2 out]
        n138 = property on="Methodenname" class="Str"("Value"=w263) -> ()  [unwired: 2 in, 2 out]
        n139 = property on="t_MainMach1" class="Arr (strict)"("Value"=w254) -> ()  [unwired: 2 in, 2 out]
        n140 = property on="T_MainMach1" class="Arr (strict)"("Value"=w253) -> ()  [unwired: 2 in, 2 out]
        n141 = property on="t_MainMach2" class="Arr (strict)"("Value"=w252) -> ()  [unwired: 2 in, 2 out]
        n142 = while {
          tunnel: w312 -> [w421]
          tunnel: w311 -> [w420]
          tunnel: w310 -> [w419]
          tunnel: w309 -> [w418]
          tunnel: w308 -> [w417]
          tunnel: w306 -> [w416]
          tunnel: w307 -> [w415]
          tunnel: w313 -> [w385]
          tunnel: [w384] -> w304
          tunnel: [w347] -> w305
          tunnel: ["EditorBeenden"] -> w303
          tunnel: w272 -> [w370]
          shift-right: [w365] -> _
          shift-left: w268 -> [w369]
          tunnel: w271 -> [w368]
          tunnel: w270 -> [w367]
          tunnel: ["AllesSpeichern"] -> w266
          tunnel: ["MethodeDuplizieren"] -> w249
          stop <- w339 stop-if-true
          n143 = for {
            tunnel: w369 -> [w430] mode=indexing
            tunnel: w370 -> [w426]
            tunnel: w368 -> [w425]
            tunnel: w367 -> [w444]
            tunnel: [w438] -> w378 mode=indexing
            n144 = Index Array(array=w430, index=0 ("Index")) -> (element=w450:dbl)
            n145 = Index Array(array=w430, index=1 ("Index")) -> (element=w448:dbl)
            n146 = Index Array(array=w430, index=3 ("Index")) -> (element=w432:dbl)
            n147 = Index Array(array=w430, index=4 ("Index")) -> (element=w431:dbl)
            n148 = Index Array(array=w430, index=6 ("Index")) -> (element=w446:dbl)
            n149 = To Long Integer(number=w450) -> (32bit integer=w449:i32)
            n150 = To Long Integer(number=w448) -> (32bit integer=w447:i32)
            n151 = To Long Integer(number=w432) -> (32bit integer=w429:i32)
            n152 = To Long Integer(number=w431) -> (32bit integer=w428:i32)
            n153 = To Long Integer(number=w446) -> (32bit integer=w445:i32)
            n154 = Index Array(array=w430, index=2 ("Index")) -> (element=w443:dbl)
            n155 = Index Array(array=w430, index=5 ("Index")) -> (element=w427:dbl)
            n156 = Index Array(array=w430, index=7 ("Index")) -> (element=w442:dbl)
            n157 = Index Array(array=w426, index=w449) -> (element=w441:string)
            n158 = Index Array(array=w425, index=w447) -> (element=w440:string)
            n159 = Index Array(array=w426, index=w429) -> (element=w424:string)
            n160 = Index Array(array=w425, index=w428) -> (element=w423:string)
            n161 = Index Array(array=w444, index=w445) -> (element=w436:string)
            n162 = Number To Exponential String(number=w443) -> (E-format string=w439:string)  [unwired: 3 in]
            n163 = Number To Exponential String(number=w427) -> (E-format string=w422:string)  [unwired: 3 in]
            n164 = Number To Exponential String(number=w442) -> (E-format string=w437:string)  [unwired: 3 in]
            n165 = Build Array(w441, w440, w439, w424, w423, w422, w436, w437) -> (w438:string[])
          }
          "ZwangsBedingungen" <- w378
          n166 = Wait (ms)(milliseconds to wait=u32 500 ("Zu wartende ms")) -> ()  [unwired: 1 out]
          n167 = Build Array("AbfragbareVariablen1", "Vergleichsoperator1", "Wert1", "AbfragbareVariablen2", "Vergleichsoperator2", "Wert2", "BedienbareVariablen", "Ausgangswert") -> (w375:dbl[])
          n168 = case shown="False" "Bedingung übernehmen" {
            tunnel: w369 -> [w460 w463]
            tunnel: w375 -> [_ w462]
            tunnel: [w460 w461] -> w376
            frame False {
            }
            frame True {
              n169 = Build Array (concatenate)(w463, w462) -> (w461:dbl[][])
            }
          }
          n170 = case shown="True" "löschen" {
            tunnel: w376 -> [w456 w459]
            tunnel: [w456 w457] -> w365
            frame False {
            }
            frame True {
              n171 = Delete From Array(array=w459, index (row)="Bedingung Nr. X") -> (array with subset deleted=w457:dbl[][])  [unwired: 2 in, 1 out]
            }
          }
          n172 = Or(x="MethodeSpeichern", y="EditorBeenden") -> (x .or. y?=w382:bool)
          n173 = Or(x=w382, y="MethodeLaden") -> (x .or. y?=w349:bool)
          n174 = local write "Zwangsbedingungen"(w365) -> ()
          n175 = Or(x=w349, y="AllesSpeichern") -> (x .or. y?=w340:bool)
          n176 = Or(x="MethodeDuplizieren", y=w340) -> (x .or. y?=w339:bool)
          n177 = Or(x="AllesSpeichern", y="MethodeSpeichern") -> (x .or. y?=w347:bool)
          n178 = Bundle("Zykluslängen [s]"="Zykluslängen [s]", "ZeitpktDIOsMod0"="ZeitpktDIOsMod0", "ZeitpktDIOsMod1"="ZeitpktDIOsMod1", "ZeitpktDIOsMod2A"="ZeitpktDIOsMod2A", "ZeitpktDIOsMod2B"="ZeitpktDIOsMod2B", "DIOsSPMod0"="DIOsSPMod0", "DIOsSPMod1"="DIOsSPMod1", "DIOsSPMod2A"="DIOsSPMod2A", "DIOsSPMod2B"="DIOsSPMod2B", "Mod0HorstZeitpkt"="Mod0HorstZeitpkt", "Mod1HorstZeitpkt"="Mod1HorstZeitpkt", "Mod2AHorstZeitpkt"="Mod2AHorstZeitpkt", "Mod2BHorstZeitpkt"="Mod2BHorstZeitpkt", "HorstSPMod0"="HorstSPMod0", "HorstSPMod1"="HorstSPMod1", "HorstSPMod2A"="HorstSPMod2A", "HorstSPMod2B"="HorstSPMod2B", "LHSetpoints"="LHSetpoints", "LHHeizen?"="LHHeizen?", "ZPktFPGABoolesch"="ZPktFPGABoolesch", "FPGABoolesch"="FPGABoolesch", "ZeitpktFPGAPID"="ZeitpktFPGAPID", "FPGAPID"="FPGAPID", "ZeitpktFPGAFixp"="ZeitpktFPGAFixp", "SHSetpoints"="SHSetpoints", "t_PreMach1"="t_PreMach1", "T_PreMach1"="T_PreMach1", "t_PreMach2"="t_PreMach2", "T_PreMach2"="T_PreMach2", "PIDs für \"träge\" Heizungen"="PIDs für \"träge\" Heizungen", "Zwangsbedingungen"="Zwangsbedingungen", "Dateien fürs MS schicken?"="Dateien fürs MS schicken?", "ZeitpunkteMPV"="ZeitpunkteMPV", "SPMPV"="SPMPV", "ZeitpktMS-1"="ZeitpktMS-1", "ZeitpktMS-2"="ZeitpktMS-2", "Int.Start1"="Int.Start1", "Int.Stop1"="Int.Stop1", "Int.Start2"="Int.Start2", "Int.Stop2"="Int.Stop2", "Methodenname"="Methodenname", "t_MainMach1"="t_MainMach1", "T_MainMach1"="T_MainMach1", "t_MainMach2"="t_MainMach2", "T_MainMach2"="T_MainMach2") -> (w384:T7)  [unwired: 1 in]
          "DIOsMod0Name" <- w385
          "DIOsMod1Name" <- w421
          "DIOsMod2AName" <- w420
          "DIOsMod2BName" <- w419
          "HorstMod0Name" <- w418
          "HorstMod2BName" <- w415
          "HorstMod2AName" <- w416
          "HorstMod1Name" <- w417
        }
        n179 = case shown="True" "MethodeLöschen" {
          tunnel: w247 -> [w314 w318]
          tunnel: [w314 w315] -> w246
          tunnel: "Methode Nummer" -> [_ w316]
          frame False {
          }
          frame True {
            n180 = invoke on="MethodeLöschen" class="Bool (strict)" method="Reinit To Default"() -> ()  [unwired: 3 in, 3 out]
            n181 = Delete From Array(array=w318, length=1, index=w316) -> (array with subset deleted=w315:T2)  [unwired: 1 out]
          }
        }
        n182 = case shown="True" w249 {
          tunnel: w246 -> [w319 w322]
          tunnel: [w319 w321] -> w250
          tunnel: "Methode Nummer" -> [_ w323]
          frame False {
          }
          frame True {
            n183 = Index Array(array=w322, index=w323) -> (element=w320:T7)
            n184 = Build Array (concatenate)(w322, w320) -> (w321:T2)
          }
        }
        n185 = case shown="True" w305 {
          tunnel: w250 -> [w332 w338]
          tunnel: w304 -> [_ w333]
          tunnel: [w332 w334] -> w265
          tunnel: "Methode Nummer" -> [_ w335]
          frame False {
          }
          frame True {
            n186 = Delete From Array(array=w338, length=1 ("Länge"), index=w335) -> (array with subset deleted=w336:T2)  [unwired: 1 out]
            n187 = Insert Into Array(array=w336, index=w335, new element=w333) -> (w334:T2)
          }
        }
        n188 = case shown="True" w266 {
          tunnel: w265 -> [_ w329]
          tunnel: w264 -> [_ w324]
          frame False {
          }
          frame True {
            n189 = Open/Create/Replace File(file path (use dialog)=w324, operation (0:open)=T6."replace" ("Operation (0:Öffnen)")) -> (refnum out=w328:refnum<file>, error out=w330:errorcluster)  [unwired: 4 in, 1 out]
            n190 = Write to Binary File(file (use dialog)=w328, data=w329, error in=w330) -> (refnum out=w326:refnum<file>, error out=w327:errorcluster)  [unwired: 3 in, 1 out]
            n191 = Close File(refnum=w326, error in=w327) -> (error out=w325:errorcluster)  [unwired: 1 out]
            n192 = call <vilib>:"Simple Error Handler.vi"("error in (no error)"=w325) -> ()  [unwired: 4 in, 5 out]
          }
        }
      }
      "Methoden" <- w216
      n193 = property on="BedienbareVariablen" class="Ring (strict)"("Strings []"=w222) -> ()  [unwired: 2 in, 2 out]
      n194 = property on="AbfragbareVariablen1" class="Ring (strict)"("Strings []"=w221) -> ()  [unwired: 2 in, 2 out]
      n195 = property on="AbfragbareVariablen2" class="Ring (strict)"("Strings []"=w221) -> ()  [unwired: 2 in, 2 out]
      n196 = property on="Vergleichsoperator1" class="Ring (strict)"("Strings []"=w220) -> ()  [unwired: 2 in, 2 out]
      "LangsameHeizungen" <- w219
    }
  }
  n197 = Close File(refnum=w19, error in=w18) -> (path=w16:path, error out=w17:errorcluster)
  n198 = call <vilib>:"Simple Error Handler.vi"("error in (no error)"=w17) -> ()  [unwired: 4 in, 5 out]
  n199 = Open/Create/Replace File(file path (use dialog)=path "C:/methoden.perx" ("Dateipfad Methoden")) -> (refnum out=w14:refnum<file>, error out=w13:errorcluster)  [unwired: 5 in, 1 out]
  n200 = Read from Binary File(5:T2 [], 8:w13, 11:w14) -> (0:w11:errorcluster, 2:w6:T2, 3:w12:refnum<file>)  [unwired: 3 in, 1 out]
  n201 = Close File(refnum=w12, error in=w11) -> (path=w9:path, error out=w10:errorcluster)
  n202 = call <vilib>:"Simple Error Handler.vi"("error in (no error)"=w10) -> ()  [unwired: 4 in, 5 out]
